vi "PV_Gnl_RunReentrantViDynamically.vi"(8 "error in":errorcluster, 11 "ViName":string) -> (0 "error out":errorcluster, 3 "ViRefNum":refnum<vi>)   [LabVIEW 2020]
doc: "Fonction :\n\nExécute un VI avec la méthode RunVI.\nCette méthode étant différente de celle qui \"appelle\" un VI tiers, ce VI possède les même différences.\nVoir l'aide sur la méthode pour plus de détails.\n\n*****\n\nEntrées : \n\nVIName : nom du VI à exécuter. Cette connexion est nécessaire.\n\nerror in : entrée d'erreur.\n\n*****\n\nSorties :\n\nVIRefNum : référence du VI exécuté.\n\nerror out : sortie d'erreur."
panel:
  # "Input"
  # "Output"
  # "Local"
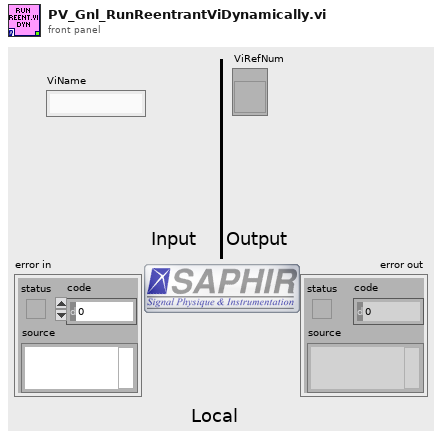
[diagram p1: front panel]
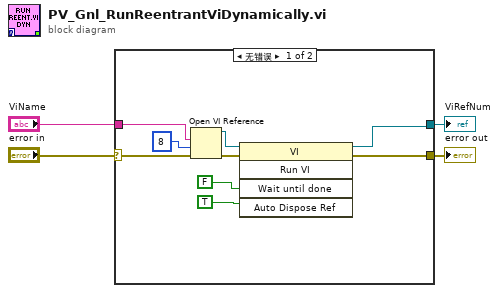
[diagram p0: block diagram]
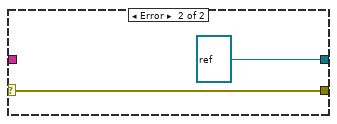
[diagram p2: hidden frame]
diagram:
  n1 = case shown="无错误" "error in" {
    selector: "error in" -> [w8 w15]
    tunnel: [w6 w15] -> w3
    tunnel: [w7 refnum<vi> refnum ("vi reference")] -> w2
    tunnel: "ViName" -> [w5 _]
    frame No Error {
      n2 = Open VI Reference(vi path=w5, options=8, error in (no error)=w8) -> (vi reference=w11:refnum<vi>, error out=w10:errorcluster)  [unwired: 3 out]
      n3 = invoke class="VI" method="Run VI"(reference=w11, error in=w10, "Wait until done"=FALSE ("Wait Until Done"), "Auto Dispose Ref"=TRUE ("Auto Dispose Reference")) -> (reference out=w7:refnum<vi>, error out=w6:errorcluster)  [unwired: 1 in, 3 out]
    }
    frame Error {
    }
  }
  "error out" <- w3
  "ViRefNum" <- w2
